vi "ifr2025 Sweep  .vi"(0 "instrument handle":refnum<visa-resource-name>, 11 "error in (no error)":errorcluster {"code" format="%.0x"}) -> (2 "Log Increment":dbl, 3 "Mode":i16, 4 "instrument handle out":refnum<visa-resource-name>, 6 "Start Frequency":dbl, 8 "Stop Frequency":dbl, 10 "Step Frequency":dbl, 12 "Type":i16, 13 "Trigger":i16, 14 "Step Time":dbl, 15 "error out":errorcluster {"code" format="%.0x"})   [LabVIEW 2009]
doc: "Returns the current sweep limits for the generator."
uses:
  Ifr2025_32.dll
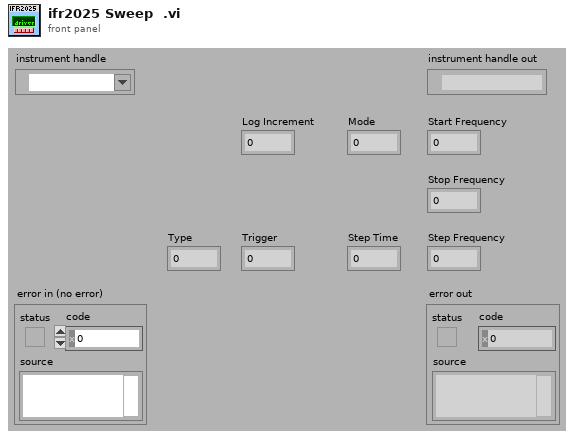
[diagram p1: front panel]
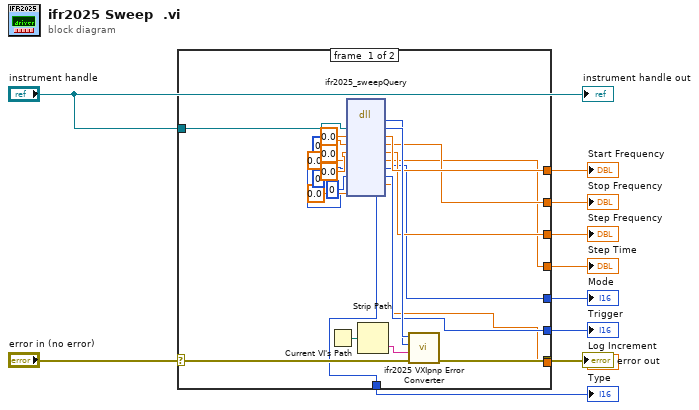
[diagram p0: block diagram]
diagram:
  n1 = case shown="No Error" "error in (no error)" {
    selector: "error in (no error)" -> [w29 w35]
    tunnel: [w28 w35] -> w11
    tunnel: "instrument handle" -> [w33 _]
    tunnel: [w26 _] -> w8
    tunnel: [w24 _] -> w7
    tunnel: [w22 _] -> w6
    tunnel: [w20 _] -> w5
    tunnel: [w18 _] -> w4
    tunnel: [w16 _] -> w3
    tunnel: [w14 _] -> w2
    tunnel: [w12 _] -> w1
    frame #0 {
      n2 = Current VI's Path() -> (path=w34:path)
      n3 = dll-call lib="P:/inst/Marconi 2024 Signal Generator/source/labview/ifr2025/ifr2025/ifr2025_*.*" fn="ifr2025_sweepQuery"("vi"=w33, "Start Frequency"=0.0, "Stop Frequency"=0.0, "Step Frequency"=0.0, "Step Time"=0.0, "Mode"=i16 0, "Trigger"=i16 0, "Log Increment"=0.0, "Type"=i16 0) -> (w31:i32, "vi"=w32:u32, "Start Frequency"=w26:dbl, "Stop Frequency"=w24:dbl, "Step Frequency"=w22:dbl, "Step Time"=w20:dbl, "Mode"=w18:i16, "Trigger"=w16:i16, "Log Increment"=w14:dbl, "Type"=w12:i16)  [unwired: 3 in, 2 out]
      n4 = Strip Path(path=w34) -> (name=w30:string)  [unwired: 1 out]
      n5 = call "ifr2025 VXIpnp Error Converter.vi"("error in (no error)"=w29, "name of VI (\"\")"=w30, "CVI error code (0)"=w31, "instrument handle"=w32) -> ("error out"=w28:errorcluster)  [unwired: 7 out]
    }
    frame #1 {
    }
  }
  "error out" <- w11
  "Start Frequency" <- w8
  "Stop Frequency" <- w7
  "Step Frequency" <- w6
  "Step Time" <- w5
  "Mode" <- w4
  "Trigger" <- w3
  "Log Increment" <- w2
  "Type" <- w1
  "instrument handle out" <- "instrument handle"
